vi "Create DM-SetPower-Command.vi"(8 "error in (no error)":errorcluster, 11 "LeftPower":dbl) -> (0 "error out":errorcluster, 3 "DM-SetPower-Command out":refnum<class "DM-SetPower-Command.lvclass">)   [LabVIEW 2013, in "DM-SetPower-Command.lvclass"]
uses:
  DM-SetPower-Command.lvclass
  DM-SetPower-Command-Arguments.ctl
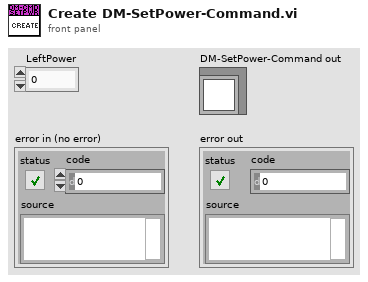
[diagram p1: front panel]
types:
  T1 = typedef "DM-SetPower-Command.lvclass/DM-SetPower-Command-Arguments.ctl" = cluster{"Power":dbl}
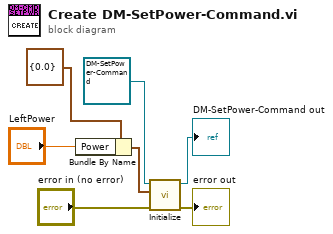
[diagram p0: block diagram]
diagram:
  n1 = Bundle By Name(cluster=T1 {"Power"=0.0} ("DM-SetPower-Command-Initialize"), "Power"="LeftPower") -> (w3:T1)
  n2 = call "Initialize.vi"("error in (no error)"="error in (no error)", "DM-SetPower-Command-Initialize"=w3, "DM-SetPower-Command in"=refnum<class "DM-SetPower-Command.lvclass"> refnum ("DM-SetPower-Command.lvclass")) -> ("error out"=→"error out":errorcluster, "DM-SetPower-Command out"=→"DM-SetPower-Command out":refnum<class "DM-SetPower-Command.lvclass">)  [unwired: 7 in]
